vi "Tell Child.vi"(4 "Priority":bool, 6 "UID":string, 7 "Actor in":refnum<class "Actor.lvclass">, 9 "Parent Stopped":bool, 10 "Safe Stop":bool=TRUE) -> (0 "Error out":errorcluster)   [LabVIEW 2025, in "jettl.lvlib" / "Stop Msg.lvlib"]
uses:
  Stop Msg.lvlib
  Actor/Actor.lvclass
  Stop Msg/Stop Msg.lvclass
  C:/git/jettl/src/jettl/jettl/Msg/Msg.lvclass
  jettl.lvlib
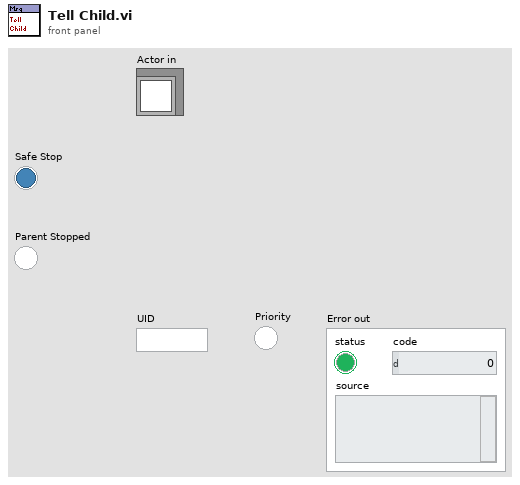
[diagram p1: front panel]
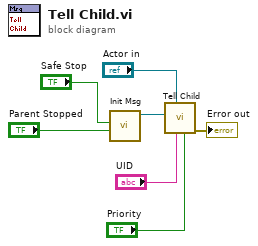
[diagram p0: block diagram]
diagram:
  n1 = call "Init Msg.vi"("Parent Stopped"="Parent Stopped", "Safe Stop"="Safe Stop") -> ("Stop Msg out"=w4:refnum<class "Stop Msg.lvclass">)  [unwired: 9 in]
  n2 = call "Tell Child.vi"("Priority"="Priority", "UID"="UID", "Actor in"="Actor in", "Msg"=w4) -> ("Error out"=→"Error out":errorcluster)  [unwired: 7 in]
